vi "Save_file.vi"(0 "Save path":path, 1 "Presure":dbl, 2 "current time":timestamp, 3 "Save":bool, 4 "Temperature":dbl, 5 "M L1 (eta1)":dbl[][](array[numeric])=[[0.0, 0.0], [0.0, 0.0], [0.0, 0.0], [0.0, 0.0], [0.0, 0.0], [0.0, 0.0]] format="%.3f", 6 "M L2 (eta2)":dbl[][](array[numeric])=[[0.0, 0.0], [0.0, 0.0], [0.0, 0.0], [0.0, 0.0], [0.0, 0.0], [0.0, 0.0]] format="%.3f", 7 "M L3 (Stereo 1)":dbl[][](array[numeric])=[[0.0, 0.0], [0.0, 0.0], [0.0, 0.0], [0.0, 0.0], [0.0, 0.0], [0.0, 0.0]] format="%.3f", 8 "M L4 (Stereo 2)":dbl[][](array[numeric])=[[0.0, 0.0], [0.0, 0.0], [0.0, 0.0], [0.0, 0.0], [0.0, 0.0], [0.0, 0.0]] format="%.3f") -> ()   [LabVIEW 2018]
uses:
  <vilib>/Utility/file.llb/Write To Spreadsheet File (string).vi
panel:
  # "IMon"
  # "VMon"
  # "IMon"
  # "VMon"
  # "IMon"
  # "VMon"
  # "IMon"
  # "VMon"
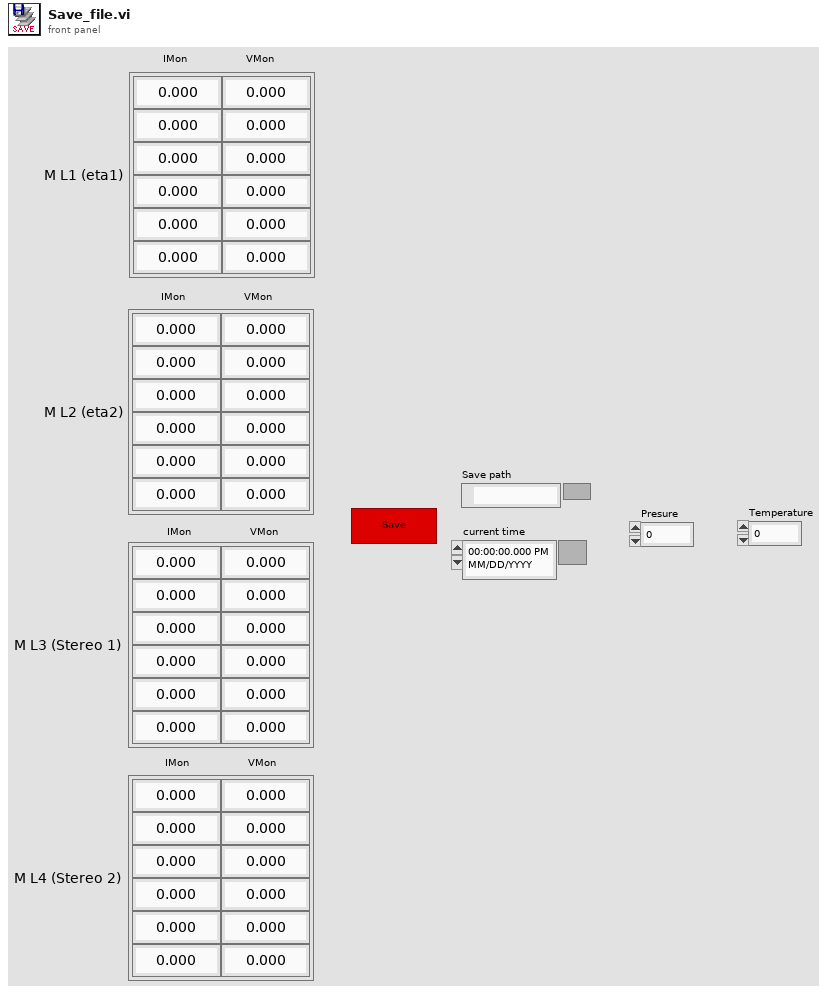
[diagram p1: front panel]
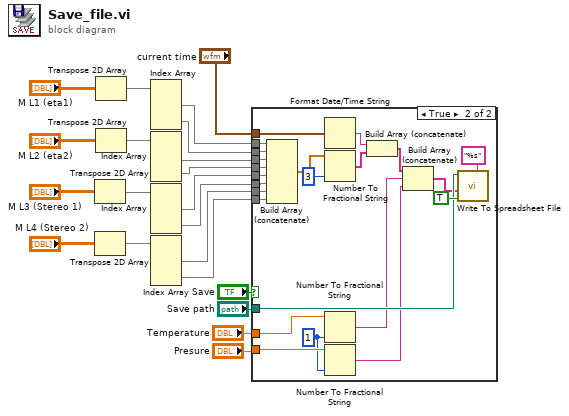
[diagram p0: block diagram]
diagram:
  n1 = Transpose 2D Array(2D array="M L3 (Stereo 1)") -> (transposed array=w12:dbl[][])
  n2 = Transpose 2D Array(2D array="M L4 (Stereo 2)") -> (transposed array=w9:dbl[][])
  n3 = Transpose 2D Array(2D array="M L1 (eta1)") -> (transposed array=w16:dbl[][])
  n4 = Transpose 2D Array(2D array="M L2 (eta2)") -> (transposed array=w14:dbl[][])
  n5 = Index Array(array=w16) -> (element #1=w8:dbl[], element #2=w7:dbl[])  [unwired: 4 in]
  n6 = Index Array(array=w14) -> (element #1=w6:dbl[], element #2=w5:dbl[])  [unwired: 4 in]
  n7 = Index Array(array=w12) -> (element #1=w4:dbl[], element #2=w3:dbl[])  [unwired: 4 in]
  n8 = Index Array(array=w9) -> (element #1=w2:dbl[], element #2=w1:dbl[])  [unwired: 4 in]
  n9 = case shown="True" "Save" {
    tunnel: "current time" -> [_ w42]
    tunnel: "Save path" -> [_ w40]
    tunnel: w8 -> [_ w38]
    tunnel: w7 -> [_ w37]
    tunnel: w6 -> [_ w36]
    tunnel: w5 -> [_ w35]
    tunnel: "Temperature" -> [_ w33]
    tunnel: "Presure" -> [_ w32]
    tunnel: w4 -> [_ w25]
    tunnel: w3 -> [_ w24]
    tunnel: w2 -> [_ w23]
    tunnel: w1 -> [_ w22]
    frame False {
    }
    frame True {
      w26 = i16 1 ("precision (6)")
      n10 = Build Array (concatenate)(w38, w37, w36, w35, w25, w24, w23, w22) -> (w34:dbl[])
      n11 = Format Date/Time String(seconds (now)=w42) -> (date/time string=w43:string)  [unwired: 2 in]
      n12 = Number To Fractional String(number=w34, precision (6)=3) -> (F-format string=w41:string[])  [unwired: 2 in]
      n13 = Number To Fractional String(number=w33, precision (6)=w26) -> (F-format string=w29:string)  [unwired: 2 in]
      n14 = Number To Fractional String(number=w32, precision (6)=w26) -> (F-format string=w28:string)  [unwired: 2 in]
      n15 = Build Array (concatenate)(w43, w41) -> (w30:string[])
      n16 = Build Array (concatenate)(w30, w29, w28) -> (w27:string[])
      n17 = call-poly <vilib>:"Write To Spreadsheet File.vi"("format (%s)"="%s", "append to file? (new file:F)"=TRUE, "1D data"=w27, "file path (dialog if empty)"=w40) -> ()  [unwired: 4 in, 1 out]
    }
  }
